vi "Self-Test.vi"(8 "error in (no error)":errorcluster, 11 "DG645 in":refnum<class "DG645.lvclass">) -> (0 "error out":errorcluster, 1 "Result Message":string, 2 "Result Code":i32, 3 "DG645 out":refnum<class "DG645.lvclass">)   [LabVIEW 2018, in "DG645.lvlib" / "DG645.lvclass"]
uses:
  DG645.lvclass
  DG645.lvclass/DG645.ctl
  <instrlib>/Stanford Research DG645/Stanford Research DG645.lvlib
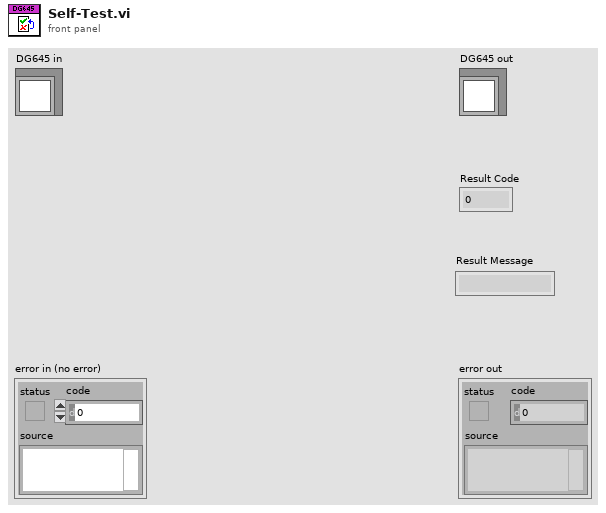
[diagram p1: front panel]
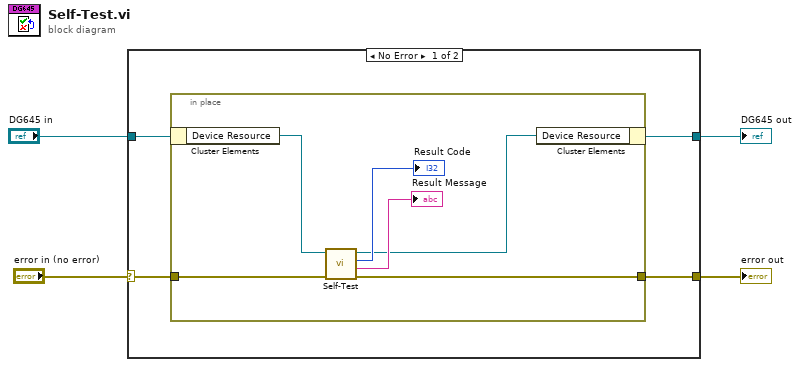
[diagram p0: block diagram]
diagram:
  n1 = case shown="No Error" "error in (no error)" {
    selector: "error in (no error)" -> [w7 w16]
    tunnel: [w6 w16] -> w3
    tunnel: [w5 w15] -> w2
    tunnel: "DG645 in" -> [w8 w15]
    frame No Error {
      n2 = in-place {
        in-place-border: w7 -> [w13]
        in-place-border: [w10] -> w6
        n3 = in-place-cluster #1(w8) -> ("Device Resource"=w14:refnum<visa-resource-name>)
        n4 = call <instrlib>:"Self-Test.vi"("error in (no error)"=w13, "VISA resource name"=w14) -> ("error out"=w10:errorcluster, "Self-Test Result Message"=→"Result Message":string, "Self-Test Result Code"=→"Result Code":i32, "VISA resource name out"=w9:refnum<visa-resource-name>)  [unwired: 6 in]
        n5 = in-place-cluster #1("Device Resource"=w9) -> (w5:refnum<class "DG645.lvclass">)
      }
    }
    frame Error {
    }
  }
  "error out" <- w3
  "DG645 out" <- w2
